vi "AVTCP-Test Data Stream.vi"() -> ()   [LabVIEW 2016]
panel:
  out "length 3":i32
  out "x-y*floor(x/y)":i32
  out "length 2":i32
  out "Array":i32[](array[numeric])
  out "last byte":u8
  out "last char":string
  out "length":i32
  in  "stop":bool
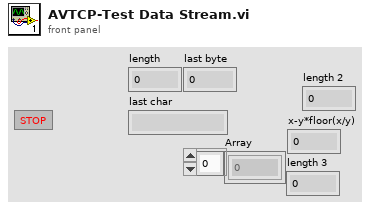
[diagram p1: front panel]
types:
  T1 = enum16{"Standard", "Buffered", "CRLF", "Immediate"}
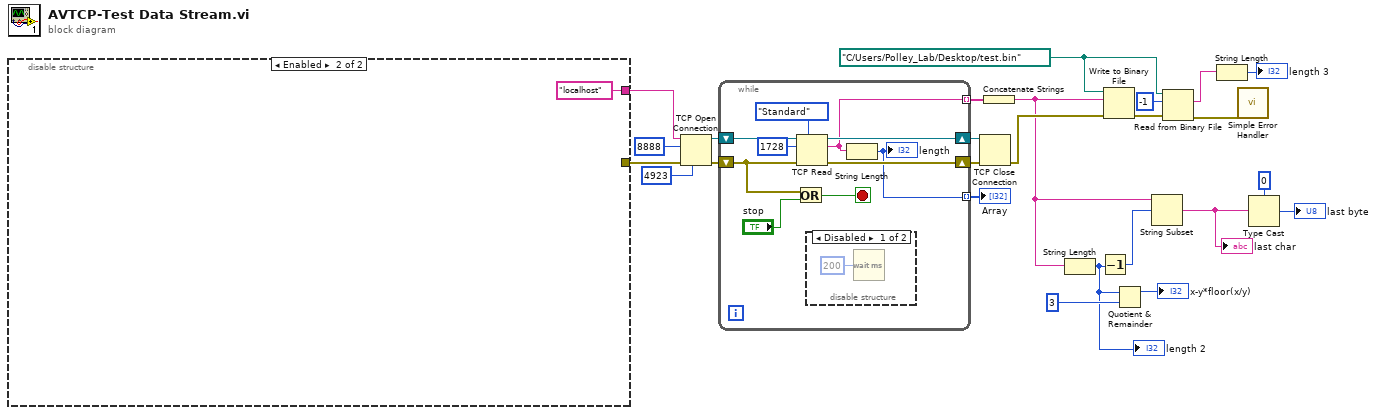
[diagram p0: block diagram]
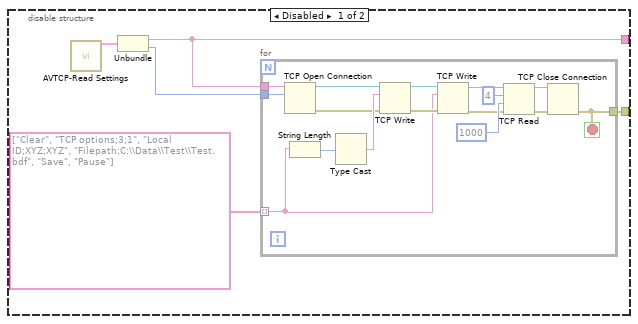
[diagram p2: hidden frame]
diagram:
  w6 = path "C:/Users/Polley_Lab/Desktop/test.bin" ("file (use dialog)")
  n1 = disable-structure shown="Enabled" {
    disable-tunnel: [w28 "localhost" ("IP Address")] -> w25
    disable-tunnel: [w26 _] -> w19
    frame Disabled {
      n2 = call "AVTCP-Read Settings.vi"() -> ("TCP"=w30:cluster{"IP Address":string, "Port":i32})  [unwired: 14 in, 1 out]
      n3 = Unbundle(w30) -> ("IP Address"=w28:string, "Port"=w27:i32)
      n4 = for {
        tunnel: string[] ["Clear", "TCP options;3;1", "Local ID;XYZ;XYZ", "Filepath;C:\\Data\\Test\\Test.bdf", "Save", "Pause"] -> [w38] mode=indexing
        tunnel: w28 -> [w37]
        tunnel: w27 -> [w36]
        tunnel: [w31] -> w26
        stop <- w31 stop-if-true
        n5 = TCP Open Connection(address=w37, remote port or service name=w36) -> (connection ID=w34:refnum<k5>, error out=w35:errorcluster)  [unwired: 3 in]
        n6 = String Length(string=w38) -> (length=w45:i32)
        n7 = Type Cast(x=w45) -> (*(type *) &x=w46:string)  [unwired: 1 in]
        n8 = TCP Write(connection ID=w34, data in=w46, error in (no error)=w35) -> (connection ID out=w43:refnum<k5>, error out=w44:errorcluster)  [unwired: 1 in, 1 out]
        n9 = TCP Write(connection ID=w43, data in=w38, error in (no error)=w44) -> (connection ID out=w40:refnum<k5>, error out=w39:errorcluster)  [unwired: 1 in, 1 out]
        n10 = TCP Read(connection ID=w40, bytes to read=4, error in (no error)=w39, 9:1000 ("timeout ms (25000)")) -> (connection ID out=w32:refnum<k5>, error out=w33:errorcluster)  [unwired: 1 in, 1 out]
        n11 = TCP Close Connection(connection ID=w32, error in (no error)=w33) -> (error out=w31:errorcluster)  [unwired: 1 in, 1 out]
      }
    }
    frame Enabled {
    }
  }
  n12 = TCP Open Connection(address=w25, remote port or service name=u16 8888, local port=u16 4923 ("local port (0)"), error in (no error)=w19) -> (connection ID=w22:refnum<k5>, error out=w23:errorcluster)  [unwired: 1 in]
  n13 = while {
    shift-right: [w54] -> w21
    shift-left: w23 -> [w55]
    shift-right: [w53] -> w20
    shift-left: w22 -> [w52]
    tunnel: [w49] -> w10 mode=indexing
    tunnel: [w48] -> w11 mode=indexing
    stop <- w56 stop-if-true
    n14 = Or(x=w55, y="stop") -> (x .or. y?=w56:bool)
    n15 = TCP Read(connection ID=w52, bytes to read=1728, error in (no error)=w55, 7:T1."Standard" ("mode (standard)")) -> (connection ID out=w53:refnum<k5>, data out=w49:string, error out=w54:errorcluster)  [unwired: 1 in]
    n16 = disable-structure shown="Disabled" {
      frame Disabled {
        n17 = Wait (ms)(milliseconds to wait=u32 200) -> ()  [unwired: 1 out]
      }
      frame Enabled {
      }
    }
    n18 = String Length(string=w49) -> (length=w48:i32)
    "length" <- w48
  }
  "Array" <- w11
  n19 = TCP Close Connection(connection ID=w20, error in (no error)=w21) -> (error out=w15:errorcluster)  [unwired: 1 in, 1 out]
  n20 = Concatenate Strings(w10) -> (w14:string)
  n21 = String Length(string=w14) -> (length=w1:i32)
  "length 2" <- w1
  n22 = Decrement(x=w1) -> (x-1=w13:i32)
  n23 = Write to Binary File(file (use dialog)=w6, data=w14, error in=w15) -> (error out=w7:errorcluster)  [unwired: 3 in, 2 out]
  n24 = Quotient & Remainder(x=w1, y=3) -> (x-y*floor(x/y)=→"x-y*floor(x/y)":i32)  [unwired: 1 out]
  n25 = String Subset(string=w14, offset (0)=w13) -> (substring=w12:string)  [unwired: 1 in]
  "last char" <- w12
  n26 = Read from Binary File(8:w7, 10:-1 ("count (1)"), 11:w6) -> (0:w5:errorcluster, 2:w4:string)  [unwired: 3 in, 2 out]
  n27 = String Length(string=w4) -> (length=→"length 3":i32)
  n28 = call <vilib>:"Simple Error Handler.vi"("error in (no error)"=w5) -> ()  [unwired: 4 in, 5 out]
  n29 = Type Cast(type=u8 0, x=w12) -> (*(type *) &x=→"last byte":u8)
